vi "Read KickY.vi"(8 "error in (no error)":errorcluster, 11 "KickToSkill in":refnum<class "KickToSkill.lvclass">) -> (0 "error out":errorcluster, 2 "KickY":dbl, 3 "KickToSkill out":refnum<class "KickToSkill.lvclass">)   [LabVIEW 2023]
uses:
  KickToSkill.lvclass
  C:/Users/ebert/Desktop/roboime/SSL_AI/Skill_class/Skill.lvclass
  C:/Users/ebert/Desktop/roboime/SSL_AI/KickToSkill_class/KickToSkill.lvclass
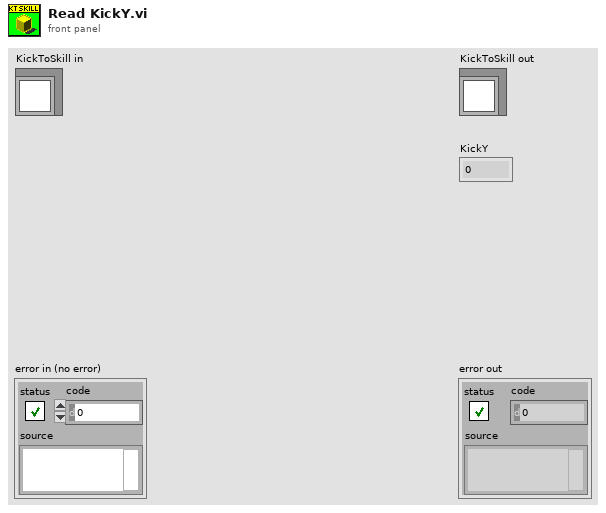
[diagram p1: front panel]
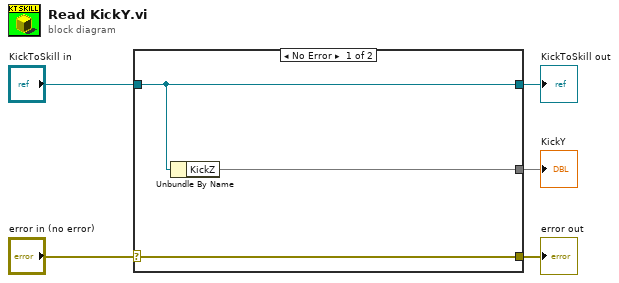
[diagram p0: block diagram]
diagram:
  n1 = case shown="No Error" "error in (no error)" {
    selector: "error in (no error)" -> [w8 w9]
    tunnel: [w8 w9] -> w4
    tunnel: [w7 w10] -> w2
    tunnel: "KickToSkill in" -> [w7 w10]
    tunnel: [w6 _] -> w1
    frame No Error {
      n2 = Unbundle By Name(w7) -> ("KickZ"=w6)
    }
    frame Error {
    }
  }
  "error out" <- w4
  "KickToSkill out" <- w2
  "KickY" <- w1
